vi "svx_Colormap Frequency In_RPM Order.vi"(7 "Frequency Type":dbl, 11 "Range":T1) -> (0 "Y":dbl[](array[numeric]), 3 "X":dbl[](array[numeric]))   [LabVIEW 2017, in "SVX Colormap.xctl"]
uses:
  <vilib>/addons/_XControls/Colormap/SVX Colormap.xctl
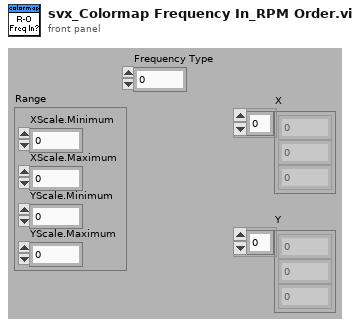
[diagram p1: front panel]
types:
  T1 = cluster{"XScale.Minimum":dbl, "XScale.Maximum":dbl, "YScale.Minimum":dbl, "YScale.Maximum":dbl}
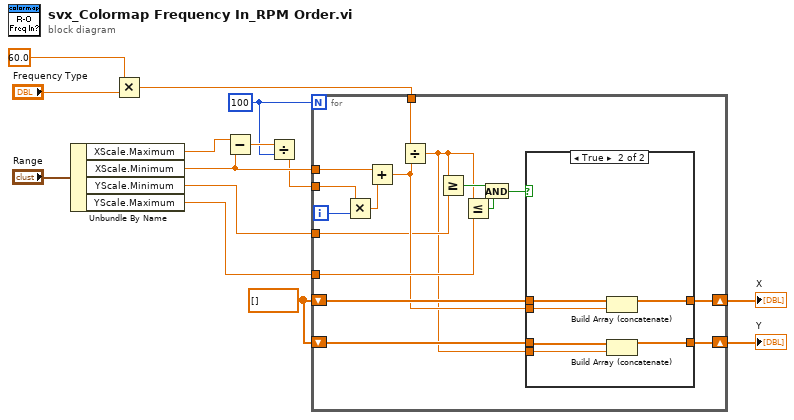
[diagram p0: block diagram]
diagram:
  w4 = 100
  w8 = dbl[] []
  n1 = Unbundle By Name("Range") -> ("XScale.Maximum"=w14:dbl, "XScale.Minimum"=w13:dbl, "YScale.Minimum"=w2:dbl, "YScale.Maximum"=w3:dbl)
  n2 = Multiply(x=60.0, y="Frequency Type") -> (x*y=w10:dbl)
  n3 = Subtract(x=w14, y=w13) -> (x-y=w9:dbl)
  n4 = Divide(x=w9, y=w4) -> (x/y=w5:dbl)
  n5 = for {
    N: w4 -> [_]
    tunnel: w5 -> [w30]
    shift-right: [w22] -> w7
    shift-left: w8 -> [w23]
    tunnel: w10 -> [w28]
    tunnel: w2 -> [w18]
    tunnel: w3 -> [w27]
    tunnel: w13 -> [w21]
    shift-right: [w16] -> w6
    shift-left: w8 -> [w17]
    i -> [w19]
    n6 = Multiply(x=w30, y=w19) -> (x*y=w29:dbl)
    n7 = Add(x=w21, y=w29) -> (x+y=w20:dbl)
    n8 = Divide(x=w28, y=w20) -> (x/y=w15:dbl)
    n9 = Greater Or Equal?(x=w15, y=w18) -> (x >= y?=w25:bool)
    n10 = Less Or Equal?(x=w15, y=w27) -> (x <= y?=w26:bool)
    n11 = And(x=w25, y=w26) -> (x .and. y?=w24:bool)
    n12 = case shown="True" w24 {
      tunnel: w23 -> [w32 w38]
      tunnel: [w32 w36] -> w22
      tunnel: w20 -> [_ w37]
      tunnel: w17 -> [w31 w35]
      tunnel: [w31 w34] -> w16
      tunnel: w15 -> [_ w33]
      frame False {
      }
      frame True {
        n13 = Build Array (concatenate)(w38, w37) -> (w36:dbl[])
        n14 = Build Array (concatenate)(w35, w33) -> (w34:dbl[])
      }
    }
  }
  "Y" <- w6
  "X" <- w7
